vi "Core1.vi"(0 "Inputs":T7, 1 "Parameters":T1, 12 "PI_Settings":T3[](array[typedef])=[{"gains"={"proportional gain"=0.0, "integral gain"=0.0}, "output range"={"output high (Inf)"=0.0, "output low (-Inf)"=0.0}, "PI_state"=enum."idle", "reset"=FALSE, "manual"=0.0}, {"gains"={"proportional gain"=0.0, "integral gain"=0.0}, "output range"={"output high (Inf)"=0.0, "output low (-Inf)"=0.0}, "PI_state"=enum."idle", "reset"=FALSE, "manual"=0.0}, {"gains"={"proportional gain"=0.0, "integral gain"=0.0}, "output range"={"output high (Inf)"=0.0, "output low (-Inf)"=0.0}, "PI_state"=enum."idle", "reset"=FALSE, "manual"=0.0}] {"gains"."proportional gain" step=0.125}) -> (4 "Outputs":T6)   [LabVIEW 2017, in "ActiveFrontEnd.lvlib"]
uses:
  ActiveFrontEnd.lvlib
  Inputs.ctl
  Outputs.ctl
  PI_Settings.ctl
  <vilib>/rvi/Analysis/control/PID/Typedef/niFpgaPID_PIGains.ctl
  <vilib>/rvi/Analysis/control/PID/Typedef/niFpgaPID_OutputRange.ctl
  Parameters.ctl
  Mode.ctl
  CascadeControlSetpt.ctl
  CascadeControlProcVar.ctl
  <userlib>/_NI FLP Library/addons/Control/Perturbance/FlpLib Perturbance 4.vi
  <userlib>/_NI FLP Library/addons/Control/Ramp/FlpLib Ramp 4.vi
  <userlib>/_NI FLP Library/FPGA/outsideSCTL/FlpLib Multiply Shared Instance 4.vi
  <userlib>/_NI FLP Library/FPGA/outsideSCTL/FlpLib Negate Outside SCTL.vi
  <userlib>/_NI FLP Library/FPGA/outsideSCTL/FlpLib Square Shared Instance 4.vi
  <userlib>/_NI FLP Library/FPGA/outsideSCTL/FlpLib Multiply Shared Instance 3.vi
  <userlib>/_NI FLP Library/FPGA/outsideSCTL/FlpLib Square Shared Instance 3.vi
  <userlib>/_NI FLP Library/FPGA/outsideSCTL/FlpLib Add Shared Instance 3.vi
  <userlib>/_NI FLP Library/FPGA/outsideSCTL/FlpLib Square Root Shared Instance 4.vi
  <userlib>/_NI FLP Library/FPGA/outsideSCTL/FlpLib Divide Shared Instance 4.vi
  <userlib>/_NI FLP Library/addons/PowerElectronics/DQtoAlphaBeta_noSine/FlpLib DQtoAlphaBeta_noSine 4.vi
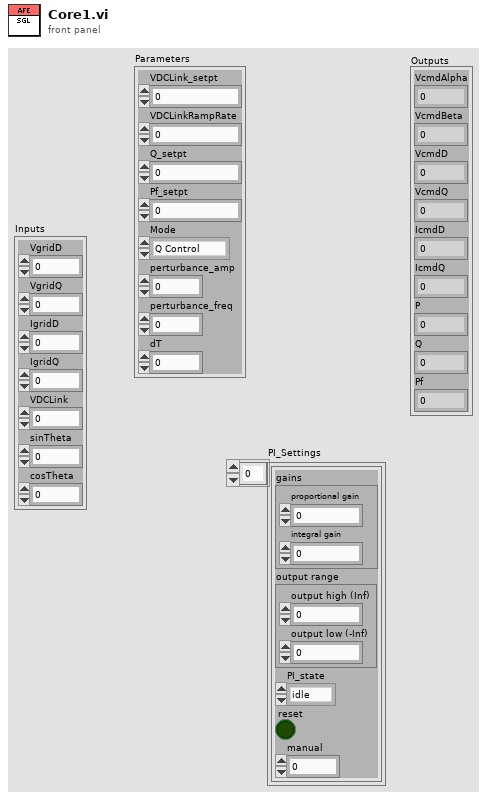
[diagram p1: front panel]
types:
  T1 = typedef "ActiveFrontEnd.lvlib/Parameters.ctl" = cluster{"VDCLink_setpt":sgl, "VDCLinkRampRate":sgl, "Q_setpt":sgl, "Pf_setpt":sgl, "Mode":T2, "perturbance_amp":sgl, "perturbance_freq":sgl, "dT":sgl}
  T2 = typedef "ActiveFrontEnd.lvlib/Mode.ctl" = enum16{"Q Control", "Pf Control"}
  T3 = typedef "ActiveFrontEnd.lvlib/PI_Settings.ctl" = cluster{"gains":T4, "output range":T5, "PI_state":enum8{"idle", "normal", "manual", "perturbance"}, "reset":bool, "manual":sgl}
  T4 = typedef "niFpgaPID_PIGains.ctl" = cluster{"proportional gain":sgl, "integral gain":sgl}
  T5 = typedef "niFpgaPID_OutputRange.ctl" = cluster{"output high (Inf)":sgl, "output low (-Inf)":sgl}
  T6 = typedef "ActiveFrontEnd.lvlib/Outputs.ctl" = cluster{"VcmdAlpha":sgl, "VcmdBeta":sgl, "VcmdD":sgl, "VcmdQ":sgl, "IcmdD":sgl, "IcmdQ":sgl, "P":sgl, "Q":sgl, "Pf":sgl}
  T7 = typedef "ActiveFrontEnd.lvlib/Inputs.ctl" = cluster{"VgridD":sgl, "VgridQ":sgl, "IgridD":sgl, "IgridQ":sgl, "VDCLink":sgl, "sinTheta":sgl, "cosTheta":sgl}
  T8 = typedef "ActiveFrontEnd.lvlib/CascadeControlProcVar.ctl" = cluster{"VDCLink":sgl, "GridVd":sgl, "GridVq":sgl, "GridId":sgl, "GridIq":sgl}
  T9 = typedef "ActiveFrontEnd.lvlib/CascadeControlSetpt.ctl" = cluster{"VDCLink":sgl, "P":sgl, "Q":sgl, "Pf":sgl}
  T10 = typedef "ActiveFrontEnd.lvlib/DQ.ctl" = cluster{"D":sgl, "Q":sgl}
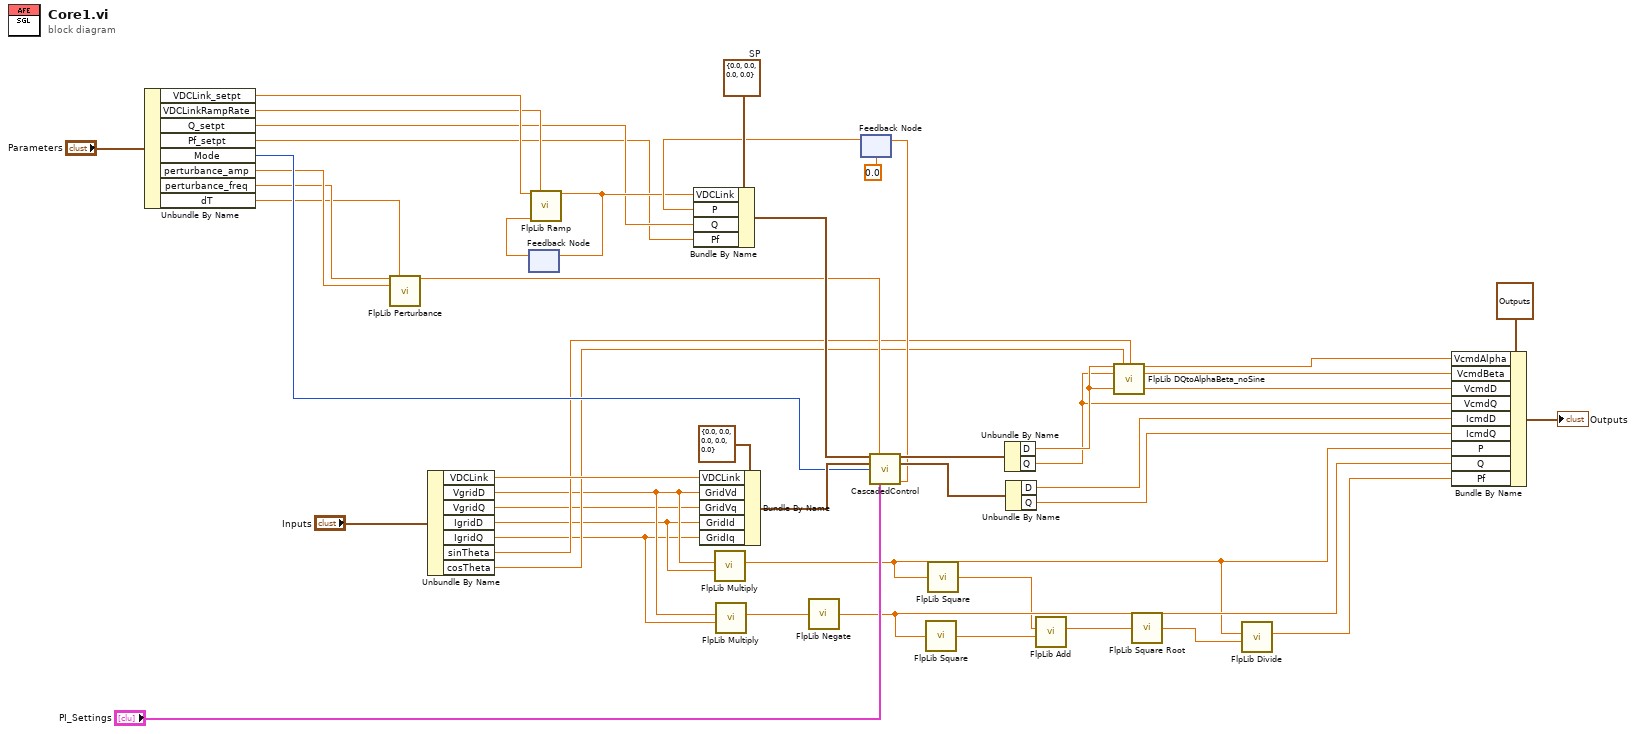
[diagram p0: block diagram]
diagram:
  w45 = T9 {"VDCLink"=0.0, "P"=0.0, "Q"=0.0, "Pf"=0.0}  # SP
  n1 = Unbundle By Name("Parameters") -> ("VDCLink_setpt"=w23:sgl, "VDCLinkRampRate"=w22:sgl, "Q_setpt"=w21:sgl, "Pf_setpt"=w20:sgl, "Mode"=w11:T2, "perturbance_amp"=w10:sgl, "perturbance_freq"=w9:sgl, "dT"=w8:sgl)
  n2 = call-poly <userlib>:"FlpLib Perturbance.vi"("freq"=w9, "dT"=w8, "amplitude"=w10) -> ("Perturbance"=w7:sgl)  [unwired: 12 in]
  n3 = Unbundle By Name("Inputs") -> ("VDCLink"=w42:sgl, "VgridD"=w4:sgl, "VgridQ"=w3:sgl, "IgridD"=w2:sgl, "IgridQ"=w1:sgl, "sinTheta"=w5:sgl, "cosTheta"=w6:sgl)
  n4 = feedback #1() -> (w32:sgl)  [unwired: 1 in]
  n5 = call-poly <userlib>:"FlpLib Ramp.vi"("input"=w23, "rampRate"=w22, "stateIn"=w32) -> ("output"=w33:sgl)  [unwired: 12 in]
  n6 = feedback-in #1(w33) -> ()
  n7 = Bundle By Name(cluster=T8 {"VDCLink"=0.0, "GridVd"=0.0, "GridVq"=0.0, "GridId"=0.0, "GridIq"=0.0} ("PV"), "VDCLink"=w42, "GridVd"=w4, "GridVq"=w3, "GridId"=w2, "GridIq"=w1) -> (w41:T8)
  n8 = call-poly <userlib>:"FlpLib Multiply.vi"("y"=w2, "x"=w4) -> ("x*y"=w14:sgl)  [unwired: 5 in]
  n9 = call-poly <userlib>:"FlpLib Multiply.vi"("y"=w1, "x"=w4) -> ("x*y"=w19:sgl)  [unwired: 5 in]
  n10 = call-poly <userlib>:"FlpLib Negate.vi"("x"=w19) -> ("-x"=w18:sgl)  [unwired: 4 in]
  n11 = feedback #2(sgl 0.0 ("Pcmd")) -> (w34:sgl)
  n12 = Bundle By Name(cluster=w45, "VDCLink"=w33, "P"=w34, "Q"=w21, "Pf"=w20) -> (w44:T9)
  n13 = call "CascadedControl.vi"("SP"=w44, "perturbance"=w7, "PV"=w41, "Mode"=w11, "PI_Settings"="PI_Settings") -> ("Vcmd"=w38:T10, "Icmd"=w37:T10, "Pcmd"=w36:sgl)  [unwired: 8 in]
  n14 = feedback-in #2(w36) -> ()
  n15 = call-poly <userlib>:"FlpLib Square.vi"("x"=w18) -> ("x^2"=w16:sgl)  [unwired: 4 in]
  n16 = call-poly <userlib>:"FlpLib Square.vi"("x"=w14) -> ("x^2"=w17:sgl)  [unwired: 4 in]
  n17 = Unbundle By Name(w38) -> ("D"=w31:sgl, "Q"=w30:sgl)
  n18 = Unbundle By Name(w37) -> ("D"=w29:sgl, "Q"=w28:sgl)
  n19 = call-poly <userlib>:"FlpLib Add.vi"("y"=w16, "x"=w17) -> ("x+y"=w15:sgl)  [unwired: 5 in]
  n20 = call-poly <userlib>:"FlpLib DQtoAlphaBeta_noSine.vi"("direct"=w31, "cosx"=w6, "sinx"=w5, "quadrature"=w30) -> ("alpha"=w27:sgl, "beta"=w26:sgl)  [unwired: 10 in]
  n21 = call-poly <userlib>:"FlpLib Square Root.vi"("x"=w15) -> ("sqrt(x)"=w13:sgl)  [unwired: 4 in]
  n22 = call-poly <userlib>:"FlpLib Divide.vi"("y"=w13, "x"=w14) -> ("x/y"=w12:sgl)  [unwired: 5 in]
  n23 = Bundle By Name(cluster=T6 {"VcmdAlpha"=0.0, "VcmdBeta"=0.0, "VcmdD"=0.0, "VcmdQ"=0.0, "IcmdD"=0.0, "IcmdQ"=0.0, "P"=0.0, "Q"=0.0, "Pf"=0.0} ("Outpus"), "VcmdAlpha"=w27, "VcmdBeta"=w26, "VcmdD"=w31, "VcmdQ"=w30, "IcmdD"=w29, "IcmdQ"=w28, "P"=w14, "Q"=w18, "Pf"=w12) -> (→"Outputs":T6)
